vi "Path Variable.vi"() -> (3 "Path Variable":string)   [LabVIEW 2019, in "SLL Environment Variable.lvlib"]
doc: "Assign <B>Path</B> as environment variable name."
uses:
  <vilib>/SLL Toolkit/SLL Environment Variable/SLL Environment Variable.lvlib
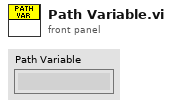
[diagram p1: front panel]
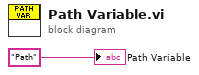
[diagram p0: block diagram]
diagram:
  "Path Variable" <- "Path" ("Name Constant")
